vi "USB Open Device.vi"(11 "DevIndex":i32) -> (3 "function return":bool)   [LabVIEW 2010, in "usb_device.lvlib"]
doc: "bool WINAPI USB_OpenDevice(int DevIndex);"
uses:
  usb_device.lvlib
  USB2XXX.dll
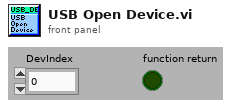
[diagram p1: front panel]
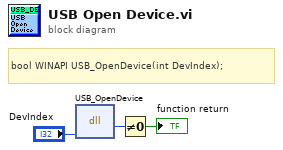
[diagram p0: block diagram]
diagram:
  # "bool WINAPI USB_OpenDevice(int DevIndex);"
  n1 = dll-call lib="G:/OtherWork/USB2XXX_Example/trunk/Labview/PublicFiles/usb_device/USB2XXX.*" fn="USB_OpenDevice"("DevIndex"="DevIndex") -> (w2:u8)  [unwired: 4 in, 2 out]
  n2 = Not Equal To 0?(x=w2) -> (x != 0?=→"function return":bool)
